vi "start twipe.vi"(8 "error in (no error)":errorcluster caption="错误输入（无错误）", 11 "HL7 输入":refnum<class "HL7.lvclass">) -> (0 "error out":errorcluster caption="错误输出", 3 "HL7 输出":refnum<class "HL7.lvclass">)   [LabVIEW 2016, in "HL7.lvlib" / "HL7.lvclass"]
uses:
  HL7.lvclass
  <vilib>/Plasmionique/MB Master/MB Master.lvlib
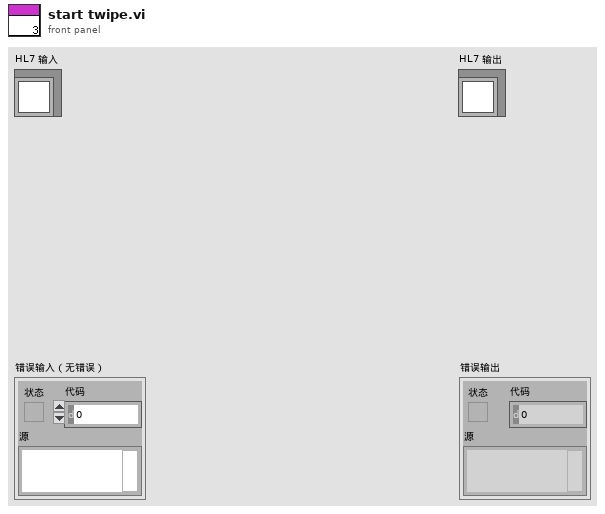
[diagram p1: front panel]
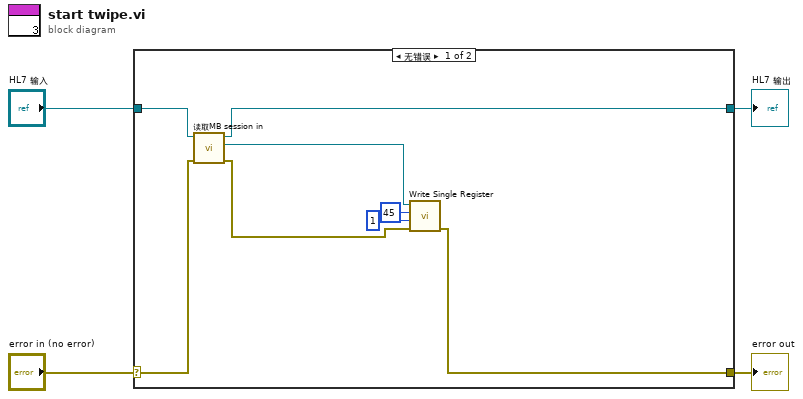
[diagram p0: block diagram]
diagram:
  n1 = case shown="无错误" "error in (no error)" {
    selector: "error in (no error)" -> [w8 w14]
    tunnel: [w6 w14] -> w3
    tunnel: [w5 w13] -> w1
    tunnel: "HL7 输入" -> [w12 w13]
    frame No Error {
      n2 = call-dynamic "读取MB session in.vi"("error in (no error)"=w8, "HL7输入"=w12) -> ("error out"=w7:errorcluster, "MB Serial Master:MB_Master"=w9:refnum<class "MB_Master.lvclass">, "HL7输出"=w5:refnum<class "HL7.lvclass">)  [unwired: 7 in]
      n3 = call <vilib>:"Write Single Register.vi"("error in (no error)"=w7, "value"=u16 1, "address"=u16 45, "MB session in"=w9) -> ("error out"=w6:errorcluster)  [unwired: 6 in, 1 out]
    }
    frame Error {
    }
  }
  "error out" <- w3
  "HL7 输出" <- w1
